vi "Stop (SILAR).vi"(3 "error in":errorcluster, 4 "Аварийная остановка":bool, 5 "Arduino Resource In":T1={"VISA resource"="", "Board Type"=enum."Uno", "Connection Type"=enum."USB / Serial", "Bytes Per Packet (15)"=15}) -> (0 "error constant out":errorcluster, 1 "Arduino Resource Out":T1={"VISA resource"="", "Board Type"=enum."Uno", "Connection Type"=enum."USB / Serial", "Bytes Per Packet (15)"=15})   [LabVIEW 2012]
uses:
  <vilib>/LabVIEW Interface for Arduino/Type Defs/Arduino Resource.ctl
  <vilib>/LabVIEW Interface for Arduino/Type Defs/Board Type.ctl
  <vilib>/LabVIEW Interface for Arduino/LabVIEW Interface for Arduino.lvlib
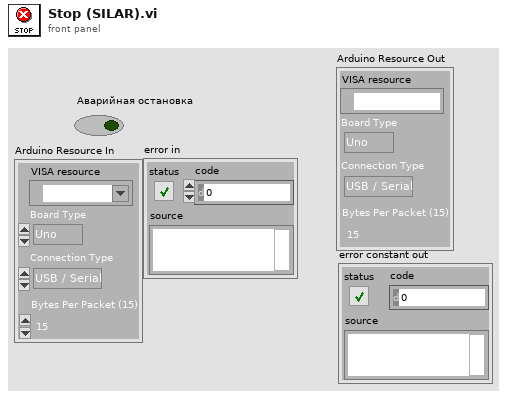
[diagram p1: front panel]
types:
  T1 = typedef "LabVIEW Interface for Arduino.lvlib/Arduino Resource.ctl" = cluster{"VISA resource":refnum<visa-resource-name>, "Board Type":T2, "Connection Type":enum8{"USB / Serial"}, "Bytes Per Packet (15)":u8}
  T2 = typedef "LabVIEW Interface for Arduino.lvlib/Board Type.ctl" = enum16{"Uno", "Dimuelanove w/Atmega 328", "Mega 2560"}
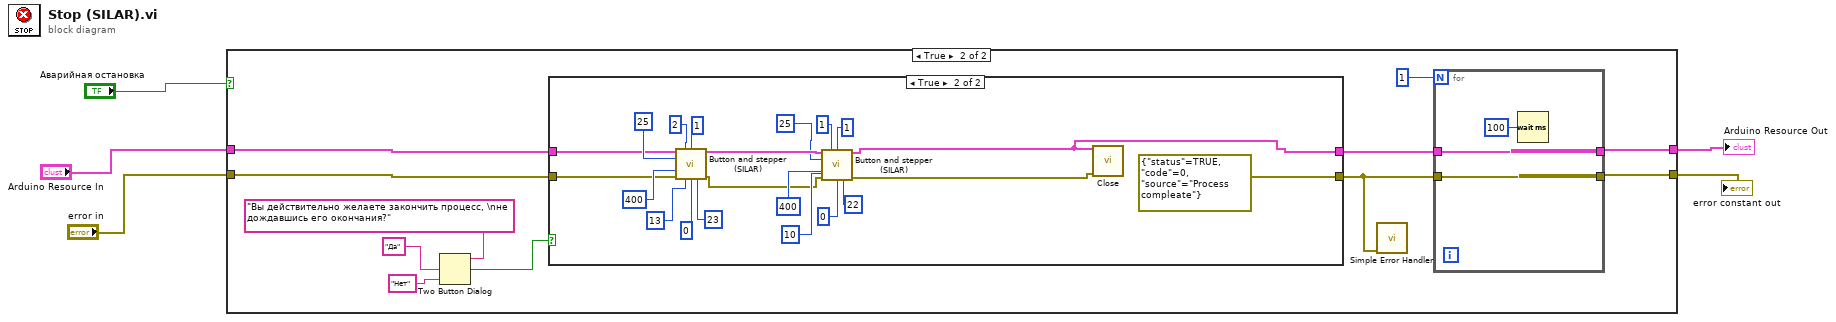
[diagram p0: block diagram]
diagram:
  n1 = case shown="True" "Аварийная остановка" {
    tunnel: "Arduino Resource In" -> [w7 w14]
    tunnel: "error in" -> [w6 w13]
    tunnel: [w7 w11] -> w2
    tunnel: [w6 w9] -> w1
    frame False {
    }
    frame True {
      n2 = Two Button Dialog(message="Вы действительно желаете закончить процесс, \nне дождавшись его окончания?", 1:"Нет" ("F button name (\"Cancel\")"), 2:"Да" ("T button name (\"OK\")")) -> (T button?=w15:bool)
      n3 = case shown="True" w15 {
        tunnel: w14 -> [w23 w28]
        tunnel: w13 -> [w22 w27]
        tunnel: [w23 w24] -> w10
        tunnel: [w22 errorcluster {"status"=TRUE, "code"=0, "source"="Process compleate"} ("error constant")] -> w8
        frame False {
        }
        frame True {
          n4 = call "Button and stepper (SILAR).vi"("Arduino Resource in"=w28, "Stepper #"=u8 2, "Turn 0n"=u8 1, "# of Steps to Move"=i16 25, "Set Speed (Steps per Second)"=i16 400, "error in"=w27, "Digital I/O Pin (0)"=u8 13, "Turn off"=u8 0, "ENABLE Pin"=u8 23) -> ("Arduino Resource out"=w44:T1, "error out"=w29:errorcluster)  [unwired: 5 in]
          n5 = call "Button and stepper (SILAR).vi"("Arduino Resource in"=w44, "Stepper #"=u8 1, "Turn 0n"=u8 1, "# of Steps to Move"=i16 25, "Set Speed (Steps per Second)"=i16 400, "error in"=w29, "Digital I/O Pin (0)"=u8 10, "Turn off"=u8 0, "ENABLE Pin"=u8 22) -> ("Arduino Resource out"=w24:T1, "error out"=w26:errorcluster)  [unwired: 5 in]
          n6 = call <vilib>:"Close.vi"("Arduino Resource"=w24, "error in"=w26) -> ()  [unwired: 13 in, 1 out]
        }
      }
      n7 = call <vilib>:"Simple Error Handler.vi"("error in (no error)"=w8) -> ()  [unwired: 4 in, 5 out]
      n8 = for {
        N: 1 -> [_]
        tunnel: [w21] -> w11
        tunnel: w10 -> [w21]
        tunnel: w8 -> [w20]
        tunnel: [w20] -> w9
        n9 = Wait (ms)(milliseconds to wait=u32 100) -> ()  [unwired: 1 out]
      }
    }
  }
  "Arduino Resource Out" <- w2
  "error constant out" <- w1
